vi "WILT Generate Initial Plot.vi"(7 "Debug":bool, 8 "Error In":errorcluster, 11 "Data File Path":path) -> (0 "Error Out":errorcluster, 3 "Mixed Signal Graph":cluster{timestamp[], "all rows":dbl[]}[](graph))   [LabVIEW 2016]
uses:
  <vilib>/Utility/file.llb/Read Delimited Spreadsheet (string).vi
  <vilib>/Utility/file.llb/Read Delimited Spreadsheet (DBL).vi
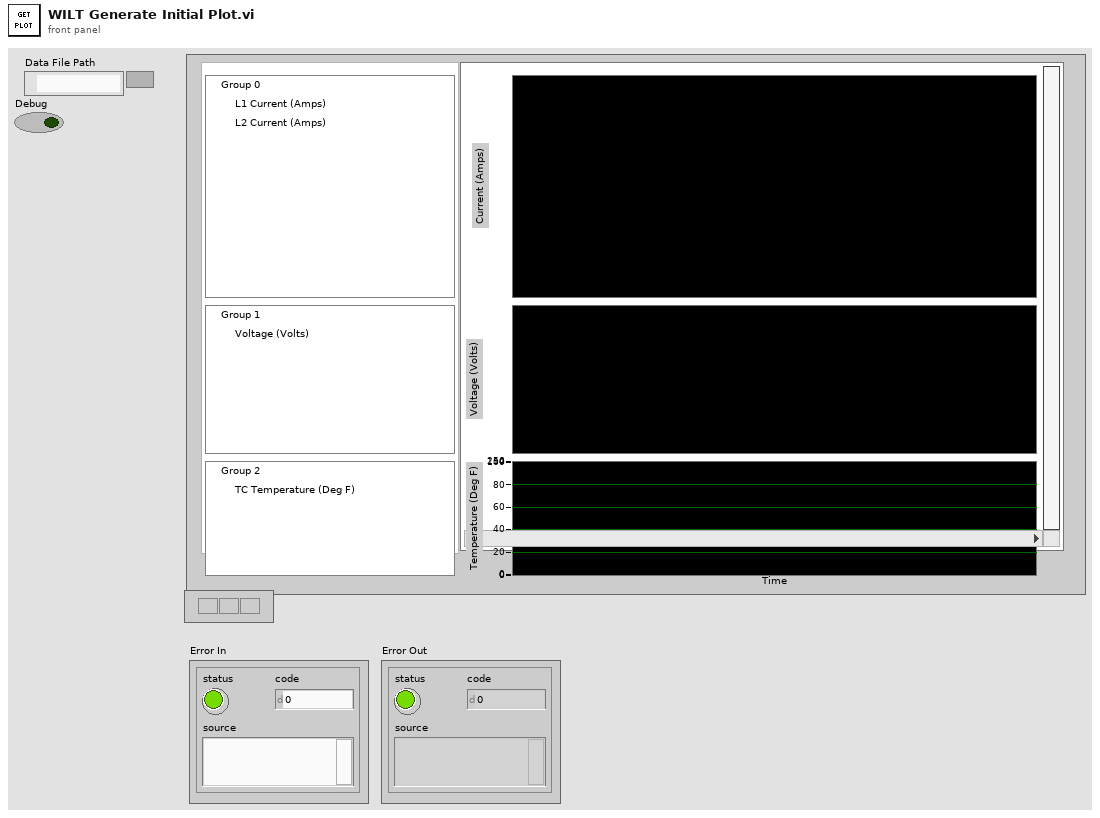
[diagram p1: front panel]
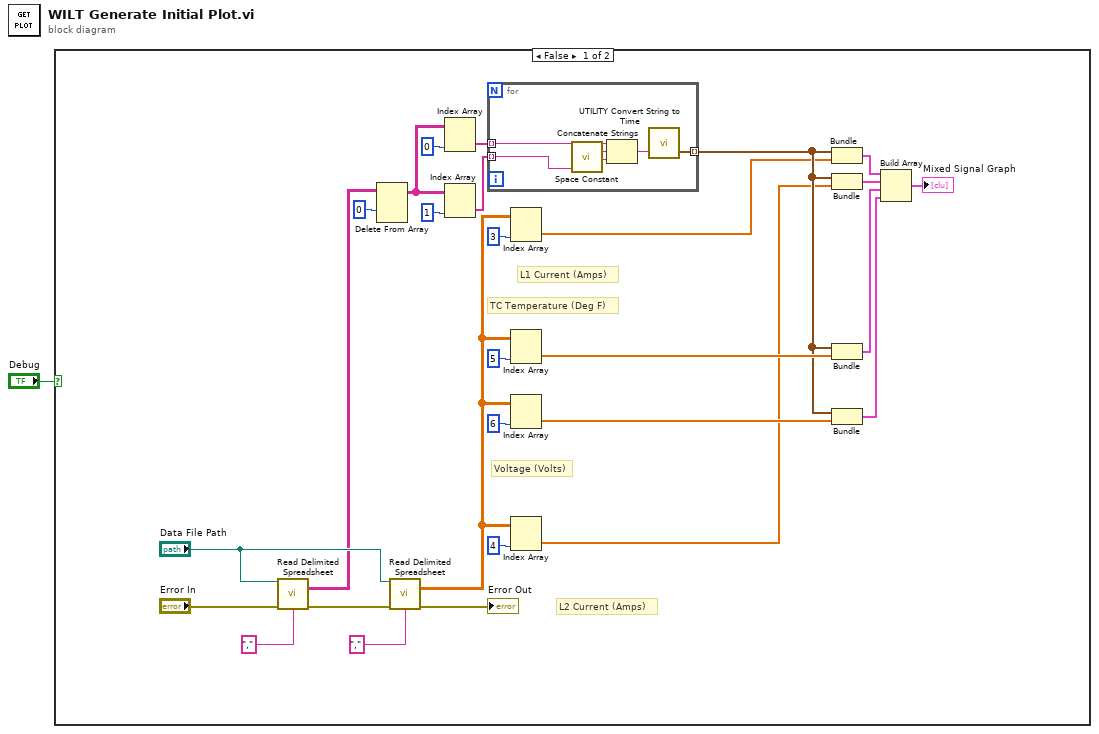
[diagram p0: block diagram]
diagram:
  n1 = case shown="False" "Debug" {
    frame False {
      # "Voltage (Volts)"
      # "TC Temperature (Deg F)"
      # "L2 Current (Amps)"
      # "L1 Current (Amps)"
      n2 = call-poly <vilib>:"Read Delimited Spreadsheet.vi"("file path (dialog if empty)"="Data File Path", "error in (no error)"="Error In", "delimiter (\\t)"="," ("delimiter (\\t)")) -> ("all rows"=w5:string[][], "error out"=w3:errorcluster)  [unwired: 7 in, 4 out]
      n3 = Delete From Array(array=w5, index (row)=0) -> (array with subset deleted=w20:string[][])  [unwired: 2 in, 1 out]
      n4 = call-poly <vilib>:"Read Delimited Spreadsheet.vi"("file path (dialog if empty)"="Data File Path", "error in (no error)"=w3, "delimiter (\\t)"="," ("delimiter (\\t)")) -> ("all rows"=w16:dbl[][], "error out"=→"Error Out":errorcluster)  [unwired: 7 in, 4 out]
      n5 = Index Array(array=w20, index (col)=0 ("disabled index (col)")) -> (element=w23:string[])  [unwired: 1 in]
      n6 = Index Array(array=w20, index (col)=1 ("disabled index (col)")) -> (element=w22:string[])  [unwired: 1 in]
      n7 = for {
        tunnel: w23 -> [w33] mode=indexing
        tunnel: w22 -> [w32] mode=indexing
        tunnel: [w30] -> w13 mode=indexing
        n8 = call <vilib>:"Space Constant.vi"() -> ("String"=w34:string)
        n9 = Concatenate Strings(w33, w34, w32) -> (w31:string)
        n10 = call "UTILITY Convert String to Time.vi"("date/time string"=w31) -> ("Resulting Time Stamp"=w30:timestamp)  [unwired: 9 in, 1 out]
      }
      n11 = Index Array(array=w16, index (col)=3) -> (element=w6:dbl[])  [unwired: 1 in]
      n12 = Index Array(array=w16, index (col)=5) -> (element=w17:dbl[])  [unwired: 1 in]
      n13 = Index Array(array=w16, index (col)=6) -> (element=w14:dbl[])  [unwired: 1 in]
      n14 = Index Array(array=w16, index (col)=4) -> (element=w7:dbl[])  [unwired: 1 in]
      n15 = Bundle(w13, "all rows"=w6) -> (w12:cluster{timestamp[], "all rows":dbl[]})  [unwired: 1 in]
      n16 = Bundle(w13, "all rows"=w7) -> (w11:cluster{timestamp[], "all rows":dbl[]})  [unwired: 1 in]
      n17 = Bundle(w13, "all rows"=w17) -> (w10:cluster{timestamp[], "all rows":dbl[]})  [unwired: 1 in]
      n18 = Bundle(w13, "all rows"=w14) -> (w9:cluster{timestamp[], "all rows":dbl[]})  [unwired: 1 in]
      n19 = Build Array(w12, w11, w10, w9) -> (→"Mixed Signal Graph":cluster{timestamp[], "all rows":dbl[]}[])
    }
    frame True {
    }
  }
